vi "Test CVT.vi"() -> ()   [LabVIEW 2014]
uses:
  <vilib>/NI/Current Value Table/DataTypes/I16_Read.vi
  <vilib>/NI/Current Value Table/DataTypes/Boolean_Read.vi
  <vilib>/NI/Current Value Table/DataTypes/Array of Single_Read.vi
  <vilib>/NI/Current Value Table/DataTypes/Array of Boolean_Read.vi
  <vilib>/NI/Current Value Table/Type to Enum.vi
  <vilib>/NI/Current Value Table/DataTypes/I16_Type To Enum.vi
  <vilib>/NI/Current Value Table/DataTypes/Boolean_Type To Enum.vi
  <vilib>/NI/Current Value Table/DataTypes/Array of Single_Type To Enum.vi
  <vilib>/NI/Current Value Table/DataTypes/Array of Boolean_Type To Enum.vi
  <vilib>/NI/Current Value Table/FGVs/CVT Globals.vi
  <vilib>/NI/Current Value Table/FGVs/Tag Memory.vi
  <vilib>/NI/Current Value Table/Memory Block.vi
  <vilib>/NI/Current Value Table/DataTypes/Boolean_Memory Block.vi
  <vilib>/NI/Current Value Table/DataTypes/Array of Boolean_Memory Block.vi
  <vilib>/NI/Current Value Table/DataTypes/Array of Single_Memory Block.vi
  <vilib>/NI/Current Value Table/DataTypes/I16_Memory Block.vi
  <vilib>/NI/Current Value Table/Current Value Table.lvlib
panel:
  out "error out":errorcluster
  out "spk.length":i16
  out "spk.period":i16
  out "spk.cycle":bool
  out "las.voffset":sgl[](array[numeric])
  out "las.vrange":sgl[](array[numeric])
  out "spk.ienabled":bool[](array[boolean])
  out "spk":bool
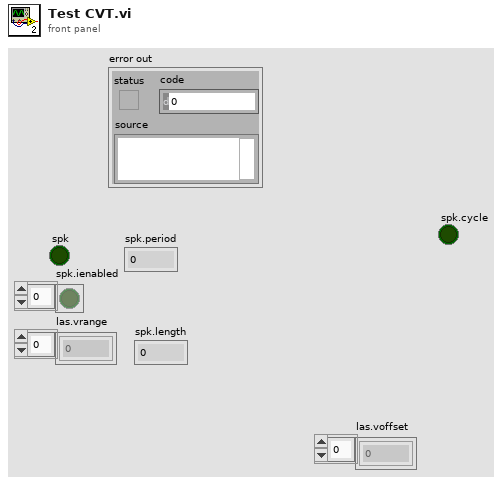
[diagram p1: front panel]
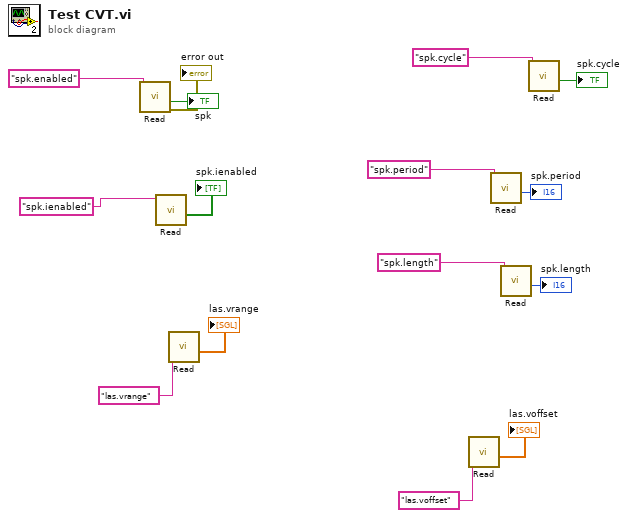
[diagram p0: block diagram]
diagram:
  n1 = call-poly <vilib>:"Read.vi"("Tag Name"="spk.enabled") -> ("error out"=→"error out":errorcluster, "Value"=→"spk":bool)  [unwired: 9 in]
  n2 = call-poly <vilib>:"Read.vi"("Tag Name"="spk.ienabled") -> ("Value"=→"spk.ienabled":bool[])  [unwired: 9 in, 1 out]
  n3 = call-poly <vilib>:"Read.vi"("Tag Name"="las.vrange") -> ("Value"=→"las.vrange":sgl[])  [unwired: 9 in, 1 out]
  n4 = call-poly <vilib>:"Read.vi"("Tag Name"="las.voffset") -> ("Value"=→"las.voffset":sgl[])  [unwired: 9 in, 1 out]
  n5 = call-poly <vilib>:"Read.vi"("Tag Name"="spk.period") -> ("Value"=→"spk.period":i16)  [unwired: 9 in, 1 out]
  n6 = call-poly <vilib>:"Read.vi"("Tag Name"="spk.length") -> ("Value"=→"spk.length":i16)  [unwired: 9 in, 1 out]
  n7 = call-poly <vilib>:"Read.vi"("Tag Name"="spk.cycle") -> ("Value"=→"spk.cycle":bool)  [unwired: 9 in, 1 out]
